vi "UDP.vi"() -> ()   [LabVIEW 2014]
panel:
  out "Resolved Color":u32 format="%.0x"
  in  "Color":bool
  in  "Color Box":u32(colorbox)
  in  "Strobe Delay":u8(slide) scale=0.0..255.0
  in  "Strobe":bool
  in  "Slide 4":u8(slide) scale=0.0..255.0
  in  "Slide 3":u8(slide) scale=0.0..255.0
  in  "Slide 2":u8(slide) scale=0.0..255.0
  in  "stop":bool
  in  "name":string
  out "data in":string caption="192.168.4.1"
  in  "port":u16
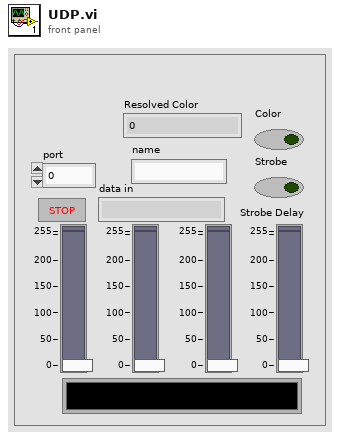
[diagram p1: front panel]
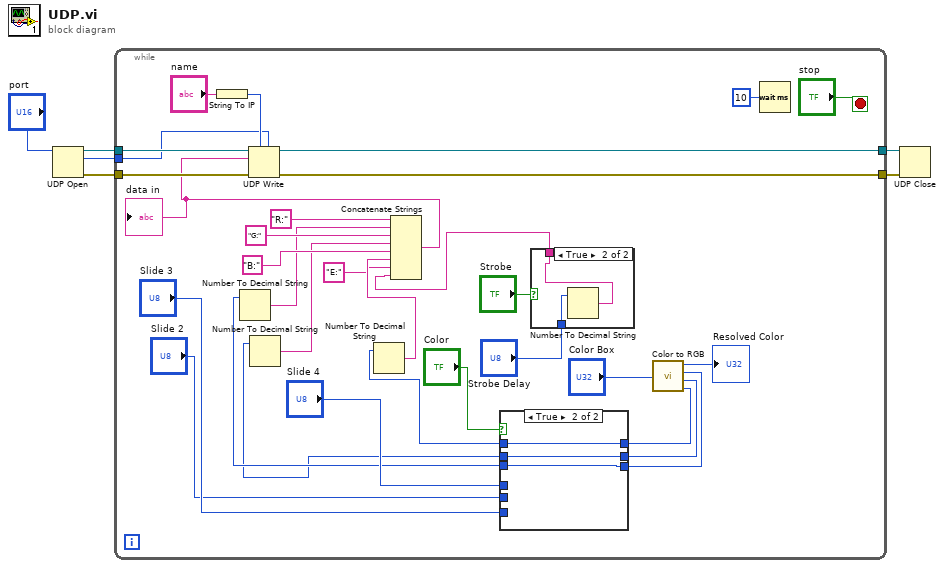
[diagram p0: block diagram]
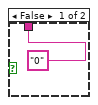
[diagram p3: hidden frame]
diagram:
  n1 = UDP Open(11:"port") -> (port=w3:refnum<k16>, 0:w1:errorcluster, 2:w2:u16)  [unwired: 4 in]
  n2 = while {
    tunnel: [w35] -> w6
    tunnel: [w34] -> w5
    tunnel: w3 -> [w33]
    tunnel: w2 -> [w32]
    tunnel: w1 -> [w31]
    stop <- "stop" stop-if-true
    n3 = String To IP(1:"name") -> (0:w37:u32)
    n4 = case shown="True" "Strobe" {
      tunnel: ["0" w47] -> w20
      tunnel: "Strobe Delay" -> [_ w46]
      frame False {
      }
      frame True {
        n5 = Number To Decimal String(number=w46) -> (decimal integer string=w47:string)  [unwired: 1 in]
      }
    }
    n6 = call <vilib>:"Color to RGB.vi"("Color"="Color Box") -> ("Resolved Color"=→"Resolved Color":u32, "R"=w8:u8, "G"=w9:u8, "B"=w10:u8)
    n7 = case shown="True" "Color" {
      tunnel: "Slide 3" -> [w41 _]
      tunnel: "Slide 2" -> [w40 _]
      tunnel: "Slide 4" -> [w39 _]
      tunnel: [w41 w42] -> w13
      tunnel: [w40 w43] -> w12
      tunnel: [w39 w44] -> w11
      tunnel: w10 -> [_ w44]
      tunnel: w9 -> [_ w43]
      tunnel: w8 -> [_ w42]
      frame False {
      }
      frame True {
      }
    }
    n8 = Number To Decimal String(number=w13) -> (decimal integer string=w26:string)  [unwired: 1 in]
    n9 = Number To Decimal String(number=w12) -> (decimal integer string=w23:string)  [unwired: 1 in]
    n10 = Number To Decimal String(number=w11) -> (decimal integer string=w29:string)  [unwired: 1 in]
    n11 = Concatenate Strings("R:", w26, "G:", w23, "B:", w29, "E:", w20) -> (w24:string)
    "data in" <- w24
    n12 = UDP Write(address=w37, port or service name=w32, connection ID=w33, data in=w24, 8:w31) -> (error out=w34:errorcluster, 3:w35:refnum<k16>)  [unwired: 1 in]
    n13 = Wait (ms)(milliseconds to wait=u32 10) -> ()  [unwired: 1 out]
  }
  n14 = UDP Close(connection ID=w6, 8:w5) -> ()  [unwired: 2 out]
